vi "TwoTanksSystem (SubVI).vi"(0 "H20 [cm]":dbl, 1 "T0 [s]":dbl=0.01, 4 "H10 [cm]":dbl, 5 "C2":dbl=32.0, 6 "C1":dbl=32.0, 7 "HLimit [cm]":dbl=40.0, 8 "qmax [cm3/s]":dbl=200.0, 9 "Valve2 On/Off":bool, 10 "Valve1 On/Off":bool, 11 "Pump On/Off":bool) -> (2 "H2 [cm]":dbl, 3 "H1 [cm]":dbl)   [LabVIEW 2020]
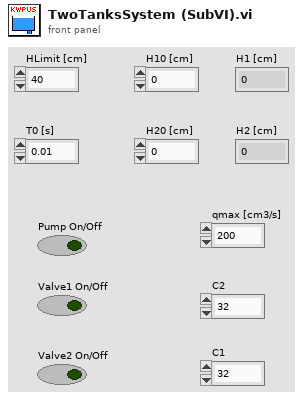
[diagram p1: front panel]
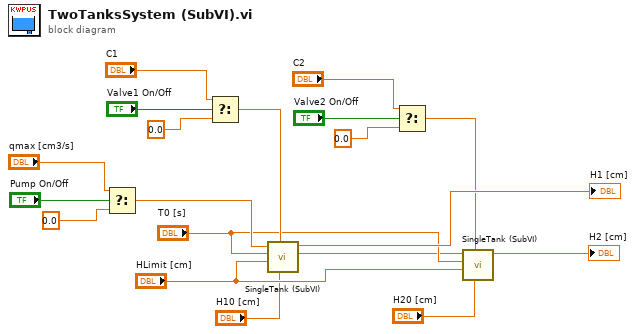
[diagram p0: block diagram]
diagram:
  n1 = Select(t="qmax [cm3/s]", s="Pump On/Off", f=0.0) -> (s? t:f=w6:dbl)
  n2 = Select(t="C1", s="Valve1 On/Off", f=0.0) -> (s? t:f=w16:dbl)
  n3 = call "SingleTank (SubVI).vi"("H0 [cm]"="H10 [cm]", "C"=w16, "HLimit [cm]"="HLimit [cm]", "T0 [s]"="T0 [s]", "q [cm3/s]"=w6) -> ("Q [cm3/s]"=w1:dbl, "H [cm]"=→"H1 [cm]":dbl)  [unwired: 5 in]
  n4 = Select(t="C2", s="Valve2 On/Off", f=0.0) -> (s? t:f=w17:dbl)
  n5 = call "SingleTank (SubVI).vi"("H0 [cm]"="H20 [cm]", "C"=w17, "HLimit [cm]"="HLimit [cm]", "T0 [s]"="T0 [s]", "q [cm3/s]"=w1) -> ("H [cm]"=→"H2 [cm]":dbl)  [unwired: 5 in, 1 out]
